vi "QMH release all.vi"(8 "error in (no error)":errorcluster, 9 "user event":refnum<user-event>, 10 "Queue in":refnum<queue>, 11 "Event Registration Refnum in":refnum<event-registration>) -> (0 "error out":errorcluster)   [LabVIEW 2020]
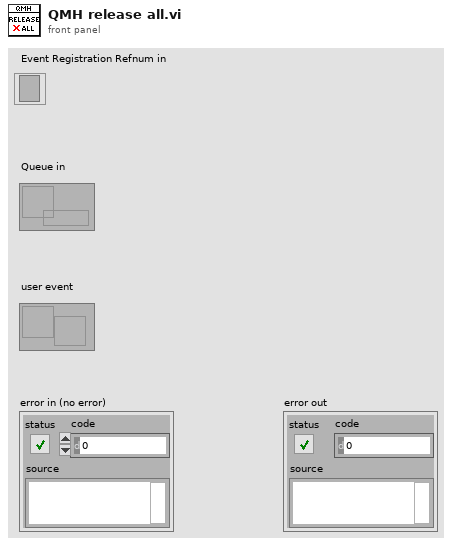
[diagram p1: front panel]
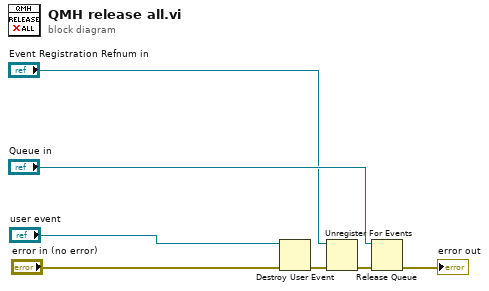
[diagram p0: block diagram]
diagram:
  n1 = Destroy User Event(user event="user event", error in="error in (no error)") -> (error out=w2:errorcluster)
  n2 = Unregister For Events(event registration refnum="Event Registration Refnum in", error in=w2) -> (error out=w5:errorcluster)
  n3 = Release Queue(queue="Queue in", error in (no error)=w5) -> (error out=→"error out":errorcluster)  [unwired: 1 in, 2 out]
